vi "Read Error data (JSON).vi"(8 "error in (no error)":errorcluster, 11 "ErrorHandler JSON in":refnum<class "ErrorHandler JSON.lvclass">) -> (0 "error out":errorcluster, 2 "Error data (JSON)":T1={"Request ID"=0, "Message type that caused error"=enum."HELLO", "Error/Abort details (JSON)"={"Error URI"="", "Error Arguments"="", "Error ArgumentKw"="{}", "Error Details"="{}"}}, 3 "ErrorHandler JSON out":refnum<class "ErrorHandler JSON.lvclass">)   [LabVIEW 2020, in "wamplv.lvlib" / "ErrorHandler JSON.lvclass"]
uses:
  ErrorHandler JSON.lvclass
  WAMP Client/API/TypeDefs/Error or abort detail (JSON).ctl
  wamplv.lvlib
  TypeDefs/WAMP Message Codes.ctl
  WAMP Client/Private/TypeDef/Error (JSON).ctl
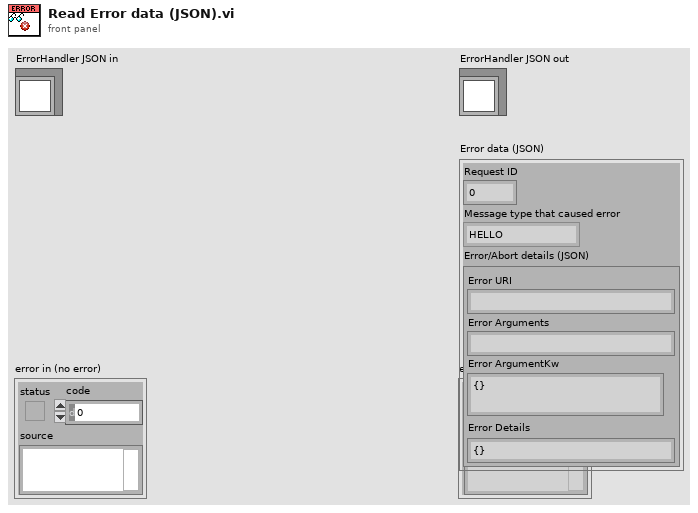
[diagram p1: front panel]
types:
  T1 = typedef "wamplv.lvlib/Error (JSON).ctl" = cluster{"Request ID":u64, "Message type that caused error":T2, "Error/Abort details (JSON)":T3}
  T2 = typedef "wamplv.lvlib/WAMP Message Codes.ctl" = enum8{"HELLO", "WELCOME", "CHALLENGE", "AUTHENTICATE", "ABORT", "GOODBYE", "ERROR", "PUBLISH", "PUBLISHED", "SUBSCRIBE", "SUBSCRIBED", "UNSUBSCRIBE", "UNSUBSCRIBED", "EVENT", "CALL", "RESULT", "REGISTER", "REGISTERED", "UNREGISTER", "UNREGISTERED", "INVOCATION", "YIELD"}
  T3 = typedef "wamplv.lvlib/Error or abort detail (JSON).ctl" = cluster{"Error URI":string, "Error Arguments":string, "Error ArgumentKw":string, "Error Details":string}
  T4 = typedef "wamplv.lvlib/Error (JSON).ctl" = cluster{"Request ID":u64, "Message type that caused error":T2, "Error/Abort details (JSON)":T5}
  T5 = typedef "wamplv.lvlib/Error or abort detail (JSON).ctl" = cluster{"Error URI":string, "Error Arguments":string, "Error ArgumentKw":string, "Error Details":string, "Associated LabVIEW Error":errorcluster}
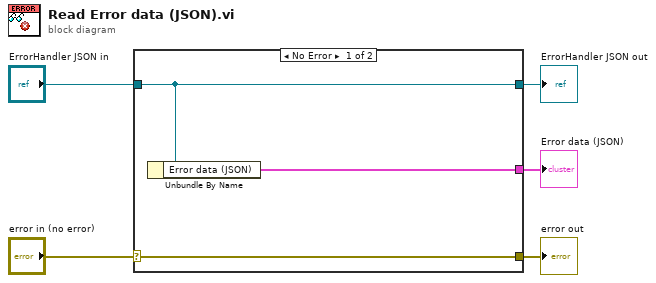
[diagram p0: block diagram]
diagram:
  n1 = case shown="No Error" "error in (no error)" {
    selector: "error in (no error)" -> [w8 w9]
    tunnel: [w8 w9] -> w4
    tunnel: [w7 w10] -> w2
    tunnel: "ErrorHandler JSON in" -> [w7 w10]
    tunnel: [w6 _] -> w1
    frame No Error {
      n2 = Unbundle By Name(w7) -> ("Error data (JSON)"=w6:T4)
    }
    frame Error {
    }
  }
  "error out" <- w4
  "ErrorHandler JSON out" <- w2
  "Error data (JSON)" <- w1
